vi "Main.vi"(7 "sweep rate, /min":dbl=0.2, 8 "sweep to:":dbl=4.0, 9 "sweep":T8(radio)=enum."2636a_smub") -> ()   [LabVIEW 2021] (continued)
                n1738 = property on="MFLI1_d3" class="Bool (strict)"() -> ("Value"=w2268:bool)  [unwired: 2 in, 2 out]
                n1739 = property on="data_caption" class="Str"() -> ("Value"=w2272:string)  [unwired: 2 in, 2 out]
                n1740 = property on="Figure_axis" class="Arr (strict)"() -> ("Value"=w2270:string[])  [unwired: 2 in, 2 out]
                n1741 = case shown="True" w2268 {
                  tunnel: w2272 -> [w2274 w2282]
                  tunnel: [w2274 w2281] -> w2271
                  tunnel: w2270 -> [w2273 w2280]
                  tunnel: [w2273 w2279] -> w2269
                  frame False {
                    # "not measure 2461 voltage (2461_meas_v)"
                  }
                  frame True {
                    w2277 = "MFLI1_d3_y"
                    w2278 = "MFLI1_d3_x"
                    w2276 = "\t"
                    w2275 = "MFLI1_d3_freq"
                    n1742 = Build Array (concatenate)(w2280, w2278, w2277, w2275) -> (w2279:string[])
                    n1743 = Concatenate Strings(w2282, w2278, w2276, w2277, w2276, w2275, w2276) -> (w2281:string)
                  }
                }
                n1744 = property on="Figure_axis" class="Arr (strict)"("Value"=w2269) -> ()  [unwired: 2 in, 2 out]
                n1745 = property on="data_caption" class="Str"("Value"=w2271) -> ()  [unwired: 2 in, 2 out]
              }
              frame #55 {
                # "MFLI_V"
                n1746 = property on="MFLI2_d3" class="Bool (strict)"() -> ("Value"=w2283:bool)  [unwired: 2 in, 2 out]
                n1747 = property on="data_caption" class="Str"() -> ("Value"=w2287:string)  [unwired: 2 in, 2 out]
                n1748 = property on="Figure_axis" class="Arr (strict)"() -> ("Value"=w2285:string[])  [unwired: 2 in, 2 out]
                n1749 = case shown="True" w2283 {
                  tunnel: w2287 -> [w2289 w2297]
                  tunnel: [w2289 w2296] -> w2286
                  tunnel: w2285 -> [w2288 w2295]
                  tunnel: [w2288 w2294] -> w2284
                  frame False {
                    # "not measure 2461 voltage (2461_meas_v)"
                  }
                  frame True {
                    w2292 = "MFLI2_d3_y"
                    w2293 = "MFLI2_d3_x"
                    w2291 = "\t"
                    w2290 = "MFLI2_d3_freq"
                    n1750 = Build Array (concatenate)(w2295, w2293, w2292, w2290) -> (w2294:string[])
                    n1751 = Concatenate Strings(w2297, w2293, w2291, w2292, w2291, w2290, w2291) -> (w2296:string)
                  }
                }
                n1752 = property on="Figure_axis" class="Arr (strict)"("Value"=w2284) -> ()  [unwired: 2 in, 2 out]
                n1753 = property on="data_caption" class="Str"("Value"=w2286) -> ()  [unwired: 2 in, 2 out]
              }
              frame #56 {
                # "MFLI_V"
                n1754 = property on="MFLI3_d3" class="Bool (strict)"() -> ("Value"=w2298:bool)  [unwired: 2 in, 2 out]
                n1755 = property on="data_caption" class="Str"() -> ("Value"=w2302:string)  [unwired: 2 in, 2 out]
                n1756 = property on="Figure_axis" class="Arr (strict)"() -> ("Value"=w2300:string[])  [unwired: 2 in, 2 out]
                n1757 = case shown="True" w2298 {
                  tunnel: w2302 -> [w2304 w2312]
                  tunnel: [w2304 w2311] -> w2301
                  tunnel: w2300 -> [w2303 w2310]
                  tunnel: [w2303 w2309] -> w2299
                  frame False {
                    # "not measure 2461 voltage (2461_meas_v)"
                  }
                  frame True {
                    w2307 = "MFLI3_d3_y"
                    w2308 = "MFLI3_d3_x"
                    w2306 = "\t"
                    w2305 = "MFLI3_d3_freq"
                    n1758 = Build Array (concatenate)(w2310, w2308, w2307, w2305) -> (w2309:string[])
                    n1759 = Concatenate Strings(w2312, w2308, w2306, w2307, w2306, w2305, w2306) -> (w2311:string)
                  }
                }
                n1760 = property on="Figure_axis" class="Arr (strict)"("Value"=w2299) -> ()  [unwired: 2 in, 2 out]
                n1761 = property on="data_caption" class="Str"("Value"=w2301) -> ()  [unwired: 2 in, 2 out]
              }
              frame #57 {
                # "MFLI_V"
                n1762 = property on="MFLI4_d3" class="Bool (strict)"() -> ("Value"=w2313:bool)  [unwired: 2 in, 2 out]
                n1763 = property on="data_caption" class="Str"() -> ("Value"=w2317:string)  [unwired: 2 in, 2 out]
                n1764 = property on="Figure_axis" class="Arr (strict)"() -> ("Value"=w2315:string[])  [unwired: 2 in, 2 out]
                n1765 = case shown="True" w2313 {
                  tunnel: w2317 -> [w2319 w2327]
                  tunnel: [w2319 w2326] -> w2316
                  tunnel: w2315 -> [w2318 w2325]
                  tunnel: [w2318 w2324] -> w2314
                  frame False {
                    # "not measure 2461 voltage (2461_meas_v)"
                  }
                  frame True {
                    w2322 = "MFLI4_d3_y"
                    w2323 = "MFLI4_d3_x"
                    w2321 = "\t"
                    w2320 = "MFLI4_d3_freq"
                    n1766 = Build Array (concatenate)(w2325, w2323, w2322, w2320) -> (w2324:string[])
                    n1767 = Concatenate Strings(w2327, w2323, w2321, w2322, w2321, w2320, w2321) -> (w2326:string)
                  }
                }
                n1768 = property on="Figure_axis" class="Arr (strict)"("Value"=w2314) -> ()  [unwired: 2 in, 2 out]
                n1769 = property on="data_caption" class="Str"("Value"=w2316) -> ()  [unwired: 2 in, 2 out]
              }
              frame #58 {
                # "MFLI_V"
                n1770 = property on="MFLI1_AuxOut0" class="Bool (strict)"() -> ("Value"=w2328:bool)  [unwired: 2 in, 2 out]
                n1771 = property on="data_caption" class="Str"() -> ("Value"=w2332:string)  [unwired: 2 in, 2 out]
                n1772 = property on="Figure_axis" class="Arr (strict)"() -> ("Value"=w2330:string[])  [unwired: 2 in, 2 out]
                n1773 = case shown="True" w2328 {
                  tunnel: w2332 -> [w2334 w2336]
                  tunnel: [w2334 w2337] -> w2331
                  tunnel: w2330 -> [w2333 w2335]
                  tunnel: [w2333 w2338] -> w2329
                  frame False {
                    # "not measure 2461 voltage (2461_meas_v)"
                  }
                  frame True {
                    w2339 = "MF1_AuxOut0"
                    n1774 = Build Array (concatenate)(w2335, w2339) -> (w2338:string[])
                    n1775 = Concatenate Strings(w2336, w2339, "\t") -> (w2337:string)
                  }
                }
                n1776 = property on="Figure_axis" class="Arr (strict)"("Value"=w2329) -> ()  [unwired: 2 in, 2 out]
                n1777 = property on="data_caption" class="Str"("Value"=w2331) -> ()  [unwired: 2 in, 2 out]
              }
            }
          }
          frame #2 {
            # "1 = 2400 1\n2 = 2400 2\n3 = 2400 3\n4 = 2636a smua\n5 = 2636a smub\n6 = do not sweep, just time\n7 = Teslatron_iPS_Field\n8 = Teslatron_iTC_Sample T"
            n1778 = property on="sweep" class="RadioBtnsControl (strict)"() -> ("Value"=w2341:T8)  [unwired: 2 in, 2 out]
            n1779 = case "reads current value from instrument which will be sweeping" shown="\"AuxOut0\"" w2341 {
              tunnel: [w2343 w2353 w2362 w2371 w2375 0.0 ("Measuremet") w2381 w2402 w2404 w2406] -> w2342
              frame "2400_1", Default {
                # "reads the voltage on 2400 1"
                n1780 = local read "2400 1 addr"() -> (w2347:u8)
                n1781 = Number To Decimal String(number=w2347) -> (decimal integer string=w2348:string)  [unwired: 1 in]
                n1782 = GPIB Write(0:w2348, 1:":READ?") -> (6:w2344:errorcluster)  [unwired: 3 in, 1 out]
                n1783 = GPIB Read(0:w2348, 1:3200, 3:w2344) -> (5:w2350:string)  [unwired: 2 in, 2 out]
                n1784 = String Subset(string=w2350, length (rest)=13) -> (substring=w2351:string)  [unwired: 1 in]
                n1785 = Fract/Exp String To Number(string=w2351) -> (number=w2343:dbl)  [unwired: 3 in, 1 out]
              }
              frame "2400_2" {
                # "reads the current on 2400 2"
                n1786 = local read "2400 2 addr"() -> (w2357:u8)
                n1787 = Number To Decimal String(number=w2357) -> (decimal integer string=w2358:string)  [unwired: 1 in]
                n1788 = GPIB Write(0:w2358, 1:":READ?") -> (6:w2354:errorcluster)  [unwired: 3 in, 1 out]
                n1789 = GPIB Read(0:w2358, 1:3200, 3:w2354) -> (5:w2360:string)  [unwired: 2 in, 2 out]
                n1790 = String Subset(string=w2360, offset (0)=14, length (rest)=13) -> (substring=w2361:string)
                n1791 = Fract/Exp String To Number(string=w2361) -> (number=w2353:dbl)  [unwired: 3 in, 1 out]
              }
              frame "2400_3" {
                # "reads the voltage on 2400 3"
                n1792 = local read "2400 3 addr"() -> (w2366:u8)
                n1793 = Number To Decimal String(number=w2366) -> (decimal integer string=w2367:string)  [unwired: 1 in]
                n1794 = GPIB Write(0:w2367, 1:":READ?") -> (6:w2363:errorcluster)  [unwired: 3 in, 1 out]
                n1795 = GPIB Read(0:w2367, 1:3200, 3:w2363) -> (5:w2369:string)  [unwired: 2 in, 2 out]
                n1796 = String Subset(string=w2369, length (rest)=13) -> (substring=w2370:string)  [unwired: 1 in]
                n1797 = Fract/Exp String To Number(string=w2370) -> (number=w2362:dbl)  [unwired: 3 in, 1 out]
              }
              frame "2636a_smua" {
                # "reads the voltage on 2636a smua"
                n1798 = local read "2614A addr"() -> (w2374:refnum<visa-resource-name>)
                n1799 = call "SinglePointMeasurement.vi"("Measure"=Measure."Voltage", "Channel"=Channel."a", "VISA resource name 2"=w2374) -> ("Measuremet"=w2371:dbl)  [unwired: 3 in, 4 out]
              }
              frame "2636a_smub" {
                # "reads the voltage on 2636a smub"
                n1800 = local read "2614A addr"() -> (w2378:refnum<visa-resource-name>)
                n1801 = call "SinglePointMeasurement.vi"("Measure"=Measure."Voltage", "Channel"=Channel."b", "VISA resource name 2"=w2378) -> ("Measuremet"=w2375:dbl)  [unwired: 3 in, 4 out]
              }
              frame "time_sweep" {
              }
              frame "iPS" {
                n1802 = property on="Sweep B" class="Bool (strict)"() -> ("Value"=w2380:bool)  [unwired: 2 in, 2 out]
                n1803 = case shown="False" w2380 {
                  tunnel: [w2382 w2400] -> w2381
                  frame False {
                    n1804 = stacked-sequence {
                      tunnel: [_ _ w2389 _] -> w2382
                      frame #0 {
                        n1805 = local read "iPS_addr_sweep"() -> (w2385:refnum<visa-resource-name>)
                        n1806 = property on="sweep to:" class="DigNum (strict)"() -> ("Value"=w2383:dbl)  [unwired: 2 in, 2 out]
                        n1807 = call "iPSset.vi"("Target Field, T"=w2383, "iPSSetCtrl"=iPSsetCtrl."Set Target Field", "VISA resource name"=w2385) -> ()  [unwired: 5 in, 4 out]
                      }
                      frame #1 {
                        n1808 = local read "iPS_addr_sweep"() -> (w2388:refnum<visa-resource-name>)
                        n1809 = property on="sweep rate, /min" class="DigNum (strict)"() -> ("Value"=w2386:dbl)  [unwired: 2 in, 2 out]
                        n1810 = call "iPSset.vi"("Field Rate, T/min"=w2386, "iPSSetCtrl"=iPSsetCtrl."Set Target Field Rate", "VISA resource name"=w2388) -> ()  [unwired: 5 in, 4 out]
                      }
                      frame #2 {
                        n1811 = property on="iPS_addr_sweep" class="VISAName"() -> ("Value"=w2391:refnum<visa-resource-name>)  [unwired: 2 in, 2 out]
                        n1812 = call "iPSread.vi"("iPSreadCtrl"=iPSreadCtrl."OutputField", "VISA resource name"=w2391) -> ("number"=w2389:dbl)  [unwired: 6 in, 3 out]
                      }
                      frame #3 {
                        n1813 = property on="sweep to:" class="DigNum (strict)"() -> ("Value"=w2392:dbl)  [unwired: 2 in, 2 out]
                        n1814 = Not Equal To 0?(x=w2392) -> (x != 0?=w2395:bool)
                        n1815 = local read "iPS_addr_sweep"() -> (w2397:refnum<visa-resource-name>)
                        n1816 = Select(t=iPSsetCtrl."Go to Field" ("iPSSetCtrl"), s=w2395, f=iPSsetCtrl."Go to Field" ("iPSSetCtrl")) -> (s? t:f=w2393:T16)
                        n1817 = call "iPSset.vi"("iPSSetCtrl"=w2393, "VISA resource name"=w2397) -> ()  [unwired: 6 in, 4 out]
                      }
                    }
                  }
                  frame True {
                    # "Measure magnetic field on IPS120-0"
                    n1818 = property on="iPS_addr_sweep" class="VISAName"() -> ("Value"=w2399:refnum<visa-resource-name>)  [unwired: 2 in, 2 out]
                    n1819 = call "iPSread.vi"("iPSreadCtrl"=iPSreadCtrl."OutputField", "VISA resource name"=w2399) -> ("number"=w2400:dbl)  [unwired: 6 in, 3 out]
                  }
                }
              }
              frame "iTC" {
                n1820 = property on="iPS_addr_sweep" class="VISAName"() -> ("Value"=w2401:refnum<visa-resource-name>)  [unwired: 2 in, 2 out]
                n1821 = call "iTCread.vi"("VISA resource name"=w2401, "iTCreadCtrl"=iTCreadCtrl."Sample Temp") -> ("number"=w2402:dbl)  [unwired: 5 in, 3 out]
              }
              frame "2461" {
                n1822 = property on="2461_addr_sweep" class="VISAName"() -> ("Value"=w2405:refnum<visa-resource-name>)  [unwired: 2 in, 2 out]
                n1823 = call <instrlib>:"Get Source Level.vi"("VISA resource name"=w2405) -> ("Current Level Out"=w2404:dbl)  [unwired: 7 in, 3 out]
              }
              frame "AuxOut0" {
                n1824 = property on="HandleOut" class="Clust (strict)"() -> ("Value"=w2408:T1)  [unwired: 2 in, 2 out]
                n1825 = call "MFLIcontrol.vi"("MFLI function"=MFLIcommand."Get AuxOut0", "handle in"=w2408) -> ("AuxOut0_Ampl"=w2406:dbl)  [unwired: 5 in, 4 out]
              }
            }
          }
          frame #3 {
            n1826 = property on="Linetrace or Mapping?" class="Bool (strict)"() -> ("Value"=w2409:bool)  [unwired: 2 in, 2 out]
            n1827 = case shown="True" w2409 {
              frame False {
                # "Reserve a name for new linetrace data file:"
                n1828 = property on="Data Folder" class="Path"() -> ("Value"=w2417:path)  [unwired: 2 in, 2 out]
                n1829 = call "AutoNamerDatExtraArtem.vi"("SweepType"="linetraces", "Custom User Path"=w2417) -> ("String"=w2415:string, "Path"=w2416:path)  [unwired: 2 in]
                n1830 = Path To String(path=w2416) -> (string=w2414:string)
                n1831 = Concatenate Strings(w2414, "\\", w2415) -> (w2413:string)
                n1832 = String To Path(string=w2413) -> (path=w2412:path)
                n1833 = local write "Data file:"(w2412) -> ()
              }
              frame True {
                n1834 = property on="Sweep Direction" class="Str"() -> ("Value"=w2418:string)  [unwired: 2 in, 2 out]
                n1835 = case shown="\"Sweep Down\"" w2418 {
                  frame "Sweep Up" {
                    n1836 = property on="UpNameString" class="Str"() -> ("Value"=w2420:string)  [unwired: 2 in, 2 out]
                    n1837 = String To Path(string=w2420) -> (path=w2419:path)
                    n1838 = local write "Data file:"(w2419) -> ()
                  }
                  frame "Sweep Down" {
                    n1839 = property on="DownNameString" class="Str"() -> ("Value"=w2421:string)  [unwired: 2 in, 2 out]
                    n1840 = String To Path(string=w2421) -> (path=w2422:path)
                    n1841 = local write "Data file:"(w2422) -> ()
                  }
                  frame "Ramp Down", Default {
                  }
                }
              }
            }
          }
          frame #4 {
            # "add \"formula\" string to the axis rings"
            n1842 = property on="Figure_axis" class="Arr (strict)"() -> ("Value"=w2425:string[])  [unwired: 2 in, 2 out]
            n1843 = Build Array (concatenate)(w2425, "formula") -> (w2423:string[])
            n1844 = property on="Figure_axis" class="Arr (strict)"("Value"=w2423) -> ()  [unwired: 2 in, 2 out]
          }
          frame #5 {
            # "passes array to ring"
            n1845 = property on="SuperHyper" class="Bool (strict)"() -> ("Value"=w2426:bool)  [unwired: 2 in, 2 out]
            n1846 = case shown="True" w2426 {
              frame True {
                # "records the fist line into the both upa nd down data file\nwhen table index=0"
                n1847 = property on="Table Index" class="DigNum (strict)"() -> ("Value"=w2435:dbl)  [unwired: 2 in, 2 out]
                n1848 = property on="HyperLoop Index" class="DigNum (strict)"() -> ("Value"=w2436:dbl)  [unwired: 2 in, 2 out]
                n1849 = property on="SuperHyper_Index" class="DigNum (strict)"() -> ("Value"=w2430:dbl)  [unwired: 2 in, 2 out]
                n1850 = Equal To 0?(x=w2435) -> (x = 0?=w2433:bool)
                n1851 = Equal To 0?(x=w2436) -> (x = 0?=w2434:bool)
                n1852 = Equal To 0?(x=w2430) -> (x = 0?=w2429:bool)
                n1853 = And(x=w2434, y=w2433) -> (x .and. y?=w2432:bool)
                n1854 = And(x=w2432, y=w2429) -> (x .and. y?=w2431:bool)
                n1855 = case shown="True" w2431 {
                  frame False {
                  }
                  frame True {
                    n1856 = property on="data_caption" class="Str"() -> ("Value"=w2440:string)  [unwired: 2 in, 2 out]
                    n1857 = local read "Data file:"() -> (w2437:path)
                    n1858 = Concatenate Strings(w2440, "\r") -> (w2439:string)
                    n1859 = Write to Text File(file (use dialog)=w2437, text=w2439) -> ()  [unwired: 2 in, 3 out]
                  }
                }
              }
              frame False {
                n1860 = property on="HyperLoop" class="Bool (strict)"() -> ("Value"=w2441:bool)  [unwired: 2 in, 2 out]
                n1861 = case shown="True" w2441 {
                  frame False {
                    n1862 = property on="Linetrace or Mapping?" class="Bool (strict)"() -> ("Value"=w2442:bool)  [unwired: 2 in, 2 out]
                    n1863 = case shown="True" w2442 {
                      frame False {
                        # "records the fist line into the data file"
                        n1864 = property on="data_caption" class="Str"() -> ("Value"=w2444:string)  [unwired: 2 in, 2 out]
                        n1865 = local read "Data file:"() -> (w2445:path)
                        n1866 = Concatenate Strings(w2444, "\r") -> (w2446:string)
                        n1867 = Write to Text File(file (use dialog)=w2445, text=w2446) -> ()  [unwired: 2 in, 3 out]
                      }
                      frame True {
                        # "records the fist line into the both upa nd down data file\nwhen table index=0"
                        n1868 = property on="Table Index" class="DigNum (strict)"() -> ("Value"=w2448:dbl)  [unwired: 2 in, 2 out]
                        n1869 = Equal To 0?(x=w2448) -> (x = 0?=w2447:bool)
                        n1870 = case shown="True" w2447 {
                          frame False {
                          }
                          frame True {
                            n1871 = property on="data_caption" class="Str"() -> ("Value"=w2452:string)  [unwired: 2 in, 2 out]
                            n1872 = local read "Data file:"() -> (w2449:path)
                            n1873 = Concatenate Strings(w2452, "\r") -> (w2451:string)
                            n1874 = Write to Text File(file (use dialog)=w2449, text=w2451) -> ()  [unwired: 2 in, 3 out]
                          }
                        }
                      }
                    }
                  }
                  frame True {
                    # "records the fist line into the both upa nd down data file\nwhen table index=0"
                    n1875 = property on="Table Index" class="DigNum (strict)"() -> ("Value"=w2456:dbl)  [unwired: 2 in, 2 out]
                    n1876 = property on="HyperLoop Index" class="DigNum (strict)"() -> ("Value"=w2457:dbl)  [unwired: 2 in, 2 out]
                    n1877 = Equal To 0?(x=w2456) -> (x = 0?=w2454:bool)
                    n1878 = Equal To 0?(x=w2457) -> (x = 0?=w2455:bool)
                    n1879 = And(x=w2455, y=w2454) -> (x .and. y?=w2453:bool)
                    n1880 = case shown="True" w2453 {
                      frame False {
                      }
                      frame True {
                        n1881 = property on="data_caption" class="Str"() -> ("Value"=w2461:string)  [unwired: 2 in, 2 out]
                        n1882 = local read "Data file:"() -> (w2458:path)
                        n1883 = Concatenate Strings(w2461, "\r") -> (w2460:string)
                        n1884 = Write to Text File(file (use dialog)=w2458, text=w2460) -> ()  [unwired: 2 in, 3 out]
                      }
                    }
                  }
                }
              }
            }
            n1885 = property on="Figure_axis" class="Arr (strict)"() -> ("Value"=w2428:string[])  [unwired: 2 in, 2 out]
            n1886 = property on="Xaxis" class="Ring (strict)"("Strings []"=w2428) -> ()  [unwired: 2 in, 2 out]
            n1887 = property on="Stop Sweep" class="Bool"("DisabledEnum"=T10."Enabled" ("Disabled")) -> ()  [unwired: 2 in, 2 out]
            n1888 = property on="Yright" class="Ring (strict)"("Strings []"=w2428) -> ()  [unwired: 2 in, 2 out]
            n1889 = property on="Yaxis" class="Ring (strict)"("Strings []"=w2428) -> ()  [unwired: 2 in, 2 out]
          }
        }
        n1890 = call "timeInSeconds.vi"() -> ("Numeric"=w1363:dbl)  [unwired: 2 in, 1 out]
        n1891 = while {
          shift-right: [w2537] -> _
          shift-left: w1362 -> [w2538]
          shift-right: [w2535] -> w1361
          shift-left: w1359 -> [w2534]
          tunnel: w1363 -> [w2532]
          stop <- w2525 stop-if-true
          # "initial value"
          # "Measure the selected channels"
          # "data array"
          # "this loop stops when target value is reached"
          # "error cluster to determine data flow"
          n1892 = stacked-sequence {
            tunnel: [_ _ w2559 _ _ _] -> w2526
            tunnel: [_ _ w2558 _ _ _] -> w2536
            tunnel: w2534 -> [_ _ w2552 _ _ _]
            tunnel: [w2544 _ _ _ _ _] -> w2533
            tunnel: w2532 -> [_ _ _ w2582 _ _]
            tunnel: [_ _ w2552 _ _ _] -> w2528
            tunnel: [_ _ _ _ _ w3348] -> w2524
            frame #0 {
              # "time is measured at the beginning\nand at the end of the cycle to\ncalculate delay time required to\nkeep set sweep rate"
              n1893 = flat-sequence {
                tunnel: [w2546] -> w2544
                frame #0 {
                  n1894 = property on="time delay, ms" class="DigNum (strict)"() -> ("Value"=w2545:dbl)  [unwired: 2 in, 2 out]
                  n1895 = Wait (ms)(milliseconds to wait=w2545) -> ()  [unwired: 1 out]
                }
                frame #1 {
                  n1896 = Tick Count (ms)() -> (millisecond timer value=w2546:u32)
                }
              }
            }
            frame #1 {
              w2547 = dbl[] []  # Empty array for data
              # "clear data array before each measurement cycle"
              n1897 = property on="data" class="Arr (strict)"("Value"=w2547) -> ()  [unwired: 2 in, 2 out]
            }
            frame #2 {
              # "add next sweep value to the data array"
              n1898 = property on="data" class="Arr (strict)"() -> ("Value"=w2557:dbl[])  [unwired: 2 in, 2 out]
              n1899 = property on="Sweep B" class="Bool (strict)"() -> ("Value"=w2549:bool)  [unwired: 2 in, 2 out]
              n1900 = local read "sweep"() -> (w2555:T8)
              n1901 = Not(x=w2549) -> (.not. x?=w2548:bool)
              n1902 = Equal?(x=w2555, y=T17."Radio Selection 7" ("sweep")) -> (x = y?=w2551:bool)
              n1903 = And(x=w2551, y=w2548) -> (x .and. y?=w2550:bool)
              n1904 = case shown="False" w2550 {
                tunnel: [w2566 w2578] -> w2559
                tunnel: [w2560 w2577] -> w2558
                tunnel: w2552 -> [_ w2575]
                tunnel: [w2560 w2575] -> w2553
                frame True {
                  n1905 = disable-structure shown="Disabled" {
                    disable-tunnel: [w2569 _] -> _
                    disable-tunnel: [w2568 _] -> _
                    frame Disabled {
                      n1906 = stacked-sequence {
                        tunnel: [_ w2571 _] -> w2569
                        tunnel: [_ _ w2573] -> w2568
                        frame #0 {
                          n1907 = local read "Hulk_SMS_addr"() -> (w2570:refnum<visa-resource-name>)
                          n1908 = VISA Clear(VISA resource name=w2570) -> ()  [unwired: 1 in, 2 out]
                        }
                        frame #1 {
                          # "acquires current output value"
                          n1909 = local read "Hulk_SMS_addr"() -> (w2572:refnum<visa-resource-name>)
                          n1910 = call "SMS_GET_OUTPUT.vi"("Hulk_SMS_addr"=w2572) -> ("Numeric"=w2571:dbl)  [unwired: 1 in, 2 out]
                        }
                        frame #2 {
                          # "checks, wheter ramp was finished"
                          n1911 = local read "Hulk_SMS_addr"() -> (w2574:refnum<visa-resource-name>)
                          n1912 = call "SMS_RAMP_STATUS.vi"("Hulk_SMS_addr"=w2574) -> ("selection"=w2573:bool)  [unwired: 1 in, 2 out]
                        }
                      }
                    }
                    frame Enabled {
                    }
                  }
                  n1913 = property on="iPS_addr_sweep" class="VISAName"() -> ("Value"=w2562:refnum<visa-resource-name>)  [unwired: 2 in, 2 out]
                  n1914 = property on="sweep to:" class="DigNum (strict)"() -> ("Value"=w2567:dbl)  [unwired: 2 in, 2 out]
                  n1915 = call "iPSread.vi"("iPSreadCtrl"=iPSreadCtrl."MagnetField", "VISA resource name"=w2562) -> ("number"=w2560:dbl)  [unwired: 6 in, 3 out]
                  n1916 = property on="Tolerance_Sweep" class="DigNum (strict)"() -> ("Value"=w2563:dbl)  [unwired: 2 in, 2 out]
                  n1917 = Subtract(x=w2560, y=w2567) -> (x-y=w2565:dbl)
                  n1918 = Absolute Value(x=w2565) -> (abs(x)=w2564:dbl)
                  n1919 = Less Or Equal?(x=w2564, y=w2563) -> (x <= y?=w2566:bool)
                }
                frame False {
                  # "calculate next value"
                  n1920 = call "CalculateNextValue.vi"("Target a 2"="sweep to:", "Channel a source value"=w2575, "Ch a sweep rate units/min"="sweep rate, /min", "time between points, sec"="time/point, sec", "Source a"=Source."Voltage") -> ("Target a"=w2577:dbl, "Boolean"=w2578:bool)
                }
              }
              n1921 = Build Array (concatenate)(w2557, w2553) -> (w2556:dbl[])
              n1922 = property on="data" class="Arr (strict)"("Value"=w2556) -> ()  [unwired: 2 in, 2 out]
            }
            frame #3 {
              n1923 = stacked-sequence "measurement sequence" {
                tunnel: w2582 -> [_ _ _ _ _ _ _ _ _ _ _ _ _ _ _ _ _ _ _ _ _ _ _ _ _ _ _ _ w2982 _ _ _ _ _ _ _ _ _ _ _ _ _ _ _ _ _ _ _ _ _ _ _ _ _ _ _ _ _ _]
                frame #0 {
                  # "check if in-phase\nsignal on lock-in 1 \nis to be measured"
                  n1924 = property on="data" class="Arr (strict)"() -> ("Value"=w2584:dbl[])  [unwired: 2 in, 2 out]
                  n1925 = local read "SR830 1 ip"() -> (w2583:bool)
                  n1926 = case shown="True" w2583 {
                    tunnel: w2584 -> [w2586 w2595]
                    tunnel: [w2586 w2594] -> w2585
                    frame False {
                      # "we are not measuring in phase signal on lock-in 1 (SR830_1_ip)"
                    }
                    frame True {
                      # "we are  measuring lock-in 1, in phase (SR830_1_ip)"
                      n1927 = local read "SR830 1 addr"() -> (w2588:u8)
                      n1928 = Number To Decimal String(number=w2588) -> (decimal integer string=w2587:string)  [unwired: 1 in]
                      n1929 = GPIB Write(0:w2587, 1:"OUTR?1") -> (6:w2593:errorcluster)  [unwired: 3 in, 1 out]
                      n1930 = GPIB Read(0:w2587, 1:3200, 3:w2593) -> (5:w2591:string)  [unwired: 2 in, 2 out]
                      n1931 = Fract/Exp String To Number(string=w2591) -> (number=w2590:dbl)  [unwired: 3 in, 1 out]
                      n1932 = Build Array (concatenate)(w2595, w2590) -> (w2594:dbl[])
                    }
                  }
                  n1933 = property on="data" class="Arr (strict)"("Value"=w2585) -> ()  [unwired: 2 in, 2 out]
                }
                frame #1 {
                  # "check if out-of-phase\nsignal on lock-in 1 \nis to be measured"
                  n1934 = property on="data" class="Arr (strict)"() -> ("Value"=w2597:dbl[])  [unwired: 2 in, 2 out]
                  n1935 = local read "SR830 1 oop"() -> (w2596:bool)
                  n1936 = case shown="True" w2596 {
                    tunnel: w2597 -> [w2599 w2608]
                    tunnel: [w2599 w2607] -> w2598
                    frame False {
                      # "we are not measuring out of phase signal on lock-in 1 (SR830_1_oop)"
                    }
                    frame True {
                      # "we are  measuring lock-in 1, out of phase (SR830_1_oop)"
                      n1937 = local read "SR830 1 addr"() -> (w2601:u8)
                      n1938 = Number To Decimal String(number=w2601) -> (decimal integer string=w2600:string)  [unwired: 1 in]
                      n1939 = GPIB Write(0:w2600, 1:"OUTR?2") -> (6:w2606:errorcluster)  [unwired: 3 in, 1 out]
                      n1940 = GPIB Read(0:w2600, 1:3200, 3:w2606) -> (5:w2604:string)  [unwired: 2 in, 2 out]
                      n1941 = Fract/Exp String To Number(string=w2604) -> (number=w2603:dbl)  [unwired: 3 in, 1 out]
                      n1942 = Build Array (concatenate)(w2608, w2603) -> (w2607:dbl[])
                    }
                  }
                  n1943 = property on="data" class="Arr (strict)"("Value"=w2598) -> ()  [unwired: 2 in, 2 out]
                }
                frame #2 {
                  # "check if in-phase\nsignal on lock-in 2 \nis to be measured"
                  n1944 = property on="data" class="Arr (strict)"() -> ("Value"=w2610:dbl[])  [unwired: 2 in, 2 out]
                  n1945 = local read "SR830 2 ip"() -> (w2609:bool)
                  n1946 = case shown="True" w2609 {
                    tunnel: w2610 -> [w2612 w2621]
                    tunnel: [w2612 w2620] -> w2611
                    frame False {
                      # "we are not measuring in phase signal on lock-in 2 (SR830_2_ip)"
                    }
                    frame True {
                      # "we are  measuring lock-in 2, in phase (SR830_2_ip)"
                      n1947 = local read "SR830 2 addr"() -> (w2614:u8)
                      n1948 = Number To Decimal String(number=w2614) -> (decimal integer string=w2613:string)  [unwired: 1 in]
                      n1949 = GPIB Write(0:w2613, 1:"OUTP?1") -> (6:w2619:errorcluster)  [unwired: 3 in, 1 out]
                      n1950 = GPIB Read(0:w2613, 1:3200, 3:w2619) -> (5:w2617:string)  [unwired: 2 in, 2 out]
                      n1951 = Fract/Exp String To Number(string=w2617) -> (number=w2616:dbl)  [unwired: 3 in, 1 out]
                      n1952 = Build Array (concatenate)(w2621, w2616) -> (w2620:dbl[])
                    }
                  }
                  n1953 = property on="data" class="Arr (strict)"("Value"=w2611) -> ()  [unwired: 2 in, 2 out]
                }
                frame #3 {
                  # "check if out-of-phase\nsignal on lock-in 2 \nis to be measured"
                  n1954 = property on="data" class="Arr (strict)"() -> ("Value"=w2623:dbl[])  [unwired: 2 in, 2 out]
                  n1955 = local read "SR830 2 oop"() -> (w2622:bool)
                  n1956 = case shown="True" w2622 {
                    tunnel: w2623 -> [w2625 w2634]
                    tunnel: [w2625 w2633] -> w2624
                    frame False {
                      # "we are not measuring out of phase signal on lock-in 2 (SR830_2_oop)"
                    }
                    frame True {
                      # "we are  measuring lock-in 2, out of phase (SR830_2_oop)"
                      n1957 = local read "SR830 2 addr"() -> (w2627:u8)
                      n1958 = Number To Decimal String(number=w2627) -> (decimal integer string=w2626:string)  [unwired: 1 in]
                      n1959 = GPIB Write(0:w2626, 1:"OUTP?2") -> (6:w2632:errorcluster)  [unwired: 3 in, 1 out]
                      n1960 = GPIB Read(0:w2626, 1:3200, 3:w2632) -> (5:w2630:string)  [unwired: 2 in, 2 out]
                      n1961 = Fract/Exp String To Number(string=w2630) -> (number=w2629:dbl)  [unwired: 3 in, 1 out]
                      n1962 = Build Array (concatenate)(w2634, w2629) -> (w2633:dbl[])
                    }
                  }
                  n1963 = property on="data" class="Arr (strict)"("Value"=w2624) -> ()  [unwired: 2 in, 2 out]
                }
                frame #4 {
                  # "check if in-phase\nsignal on lock-in 3 \nis to be measured"
                  n1964 = property on="data" class="Arr (strict)"() -> ("Value"=w2636:dbl[])  [unwired: 2 in, 2 out]
                  n1965 = local read "SR830 3 ip"() -> (w2635:bool)
                  n1966 = case shown="True" w2635 {
                    tunnel: w2636 -> [w2638 w2647]
                    tunnel: [w2638 w2646] -> w2637
                    frame False {
                      # "we are not measuring in phase signal on lock-in 3 (SR830_3_ip)"
                    }
                    frame True {
                      # "we are  measuring lock-in 3, in phase (SR830_3_ip)"
                      n1967 = local read "SR830 3 addr"() -> (w2640:u8)
                      n1968 = Number To Decimal String(number=w2640) -> (decimal integer string=w2639:string)  [unwired: 1 in]
                      n1969 = GPIB Write(0:w2639, 1:"OUTP?1") -> (6:w2645:errorcluster)  [unwired: 3 in, 1 out]
                      n1970 = GPIB Read(0:w2639, 1:3200, 3:w2645) -> (5:w2643:string)  [unwired: 2 in, 2 out]
                      n1971 = Fract/Exp String To Number(string=w2643) -> (number=w2642:dbl)  [unwired: 3 in, 1 out]
                      n1972 = Build Array (concatenate)(w2647, w2642) -> (w2646:dbl[])
                    }
                  }
                  n1973 = property on="data" class="Arr (strict)"("Value"=w2637) -> ()  [unwired: 2 in, 2 out]
                }
                frame #5 {
                  # "check if out-of-phase\nsignal on lock-in 3 \nis to be measured"
                  n1974 = property on="data" class="Arr (strict)"() -> ("Value"=w2649:dbl[])  [unwired: 2 in, 2 out]
                  n1975 = local read "SR830 3 oop"() -> (w2648:bool)
                  n1976 = case shown="True" w2648 {
                    tunnel: w2649 -> [w2651 w2660]
                    tunnel: [w2651 w2659] -> w2650
                    frame False {
                      # "we are not measuring out of phase signal on lock-in 3 (SR830_3_oop)"
                    }
                    frame True {
                      # "we are  measuring lock-in 3, out of phase (SR830_3_oop)"
                      n1977 = local read "SR830 3 addr"() -> (w2653:u8)
                      n1978 = Number To Decimal String(number=w2653) -> (decimal integer string=w2652:string)  [unwired: 1 in]
                      n1979 = GPIB Write(0:w2652, 1:"OUTP?2") -> (6:w2658:errorcluster)  [unwired: 3 in, 1 out]
                      n1980 = GPIB Read(0:w2652, 1:3200, 3:w2658) -> (5:w2656:string)  [unwired: 2 in, 2 out]
                      n1981 = Fract/Exp String To Number(string=w2656) -> (number=w2655:dbl)  [unwired: 3 in, 1 out]
                      n1982 = Build Array (concatenate)(w2660, w2655) -> (w2659:dbl[])
                    }
                  }
                  n1983 = property on="data" class="Arr (strict)"("Value"=w2650) -> ()  [unwired: 2 in, 2 out]
                }
                frame #6 {
                  # "check if in-phase\nsignal on lock-in 4 \nis to be measured"
                  n1984 = property on="data" class="Arr (strict)"() -> ("Value"=w2662:dbl[])  [unwired: 2 in, 2 out]
                  n1985 = local read "SR830 4 ip"() -> (w2661:bool)
                  n1986 = case shown="True" w2661 {
                    tunnel: w2662 -> [w2664 w2673]
                    tunnel: [w2664 w2672] -> w2663
                    frame False {
                      # "we are not measuring in phase signal on lock-in 4 (SR830_4_ip)"
                    }
                    frame True {
                      # "we are  measuring lock-in 4, in phase (SR830_4_ip)"
                      n1987 = local read "SR830 4 addr"() -> (w2666:u8)
                      n1988 = Number To Decimal String(number=w2666) -> (decimal integer string=w2665:string)  [unwired: 1 in]
                      n1989 = GPIB Write(0:w2665, 1:"OUTP?1") -> (6:w2671:errorcluster)  [unwired: 3 in, 1 out]
                      n1990 = GPIB Read(0:w2665, 1:3200, 3:w2671) -> (5:w2669:string)  [unwired: 2 in, 2 out]
                      n1991 = Fract/Exp String To Number(string=w2669) -> (number=w2668:dbl)  [unwired: 3 in, 1 out]
                      n1992 = Build Array (concatenate)(w2673, w2668) -> (w2672:dbl[])
                    }
                  }
                  n1993 = property on="data" class="Arr (strict)"("Value"=w2663) -> ()  [unwired: 2 in, 2 out]
                }
                frame #7 {
                  # "check if out-of-phase\nsignal on lock-in 4 \nis to be measured"
                  n1994 = property on="data" class="Arr (strict)"() -> ("Value"=w2675:dbl[])  [unwired: 2 in, 2 out]
                  n1995 = local read "SR830 4 oop"() -> (w2674:bool)
                  n1996 = case shown="True" w2674 {
                    tunnel: w2675 -> [w2677 w2686]
                    tunnel: [w2677 w2685] -> w2676
                    frame False {
                      # "we are not measuring out of phase signal on lock-in 4 (SR830_4_oop)"
                    }
                    frame True {
                      # "we are  measuring lock-in 4, out of phase (SR830_4_oop)"
                      n1997 = local read "SR830 4 addr"() -> (w2679:u8)
                      n1998 = Number To Decimal String(number=w2679) -> (decimal integer string=w2678:string)  [unwired: 1 in]
                      n1999 = GPIB Write(0:w2678, 1:"OUTP?2") -> (6:w2684:errorcluster)  [unwired: 3 in, 1 out]
                      n2000 = GPIB Read(0:w2678, 1:3200, 3:w2684) -> (5:w2682:string)  [unwired: 2 in, 2 out]
                      n2001 = Fract/Exp String To Number(string=w2682) -> (number=w2681:dbl)  [unwired: 3 in, 1 out]
                      n2002 = Build Array (concatenate)(w2686, w2681) -> (w2685:dbl[])
                    }
                  }
                  n2003 = property on="data" class="Arr (strict)"("Value"=w2676) -> ()  [unwired: 2 in, 2 out]
                }
                frame #8 {
                  # "check if in-phase\nsignal on lock-in 5 \nis to be measured"
                  n2004 = property on="data" class="Arr (strict)"() -> ("Value"=w2688:dbl[])  [unwired: 2 in, 2 out]
                  n2005 = local read "SR830 5 ip"() -> (w2687:bool)
                  n2006 = case shown="True" w2687 {
                    tunnel: w2688 -> [w2690 w2699]
                    tunnel: [w2690 w2698] -> w2689
                    frame False {
                      # "we are not measuring in phase signal on lock-in 5 (SR830_5_ip)"
                    }
                    frame True {
                      # "we are  measuring lock-in 5 in phase (SR830_5_ip)"
                      n2007 = local read "SR830 5 addr"() -> (w2692:u8)
                      n2008 = Number To Decimal String(number=w2692) -> (decimal integer string=w2691:string)  [unwired: 1 in]
                      n2009 = GPIB Write(0:w2691, 1:"OUTP?1") -> (6:w2697:errorcluster)  [unwired: 3 in, 1 out]
                      n2010 = GPIB Read(0:w2691, 1:3200, 3:w2697) -> (5:w2695:string)  [unwired: 2 in, 2 out]
                      n2011 = Fract/Exp String To Number(string=w2695) -> (number=w2694:dbl)  [unwired: 3 in, 1 out]
                      n2012 = Build Array (concatenate)(w2699, w2694) -> (w2698:dbl[])
                    }
                  }
                  n2013 = property on="data" class="Arr (strict)"("Value"=w2689) -> ()  [unwired: 2 in, 2 out]
                }
                frame #9 {
                  # "check if out-of-phase\nsignal on lock-in 5 \nis to be measured"
                  n2014 = property on="data" class="Arr (strict)"() -> ("Value"=w2701:dbl[])  [unwired: 2 in, 2 out]
                  n2015 = local read "SR830 5 oop"() -> (w2700:bool)
                  n2016 = case shown="True" w2700 {
                    tunnel: w2701 -> [w2703 w2712]
                    tunnel: [w2703 w2711] -> w2702
                    frame False {
                      # "we are not measuring out of phase signal on lock-in 5 (SR830_5_oop)"
                    }
                    frame True {
                      # "we are  measuring lock-in 5 out of phase (SR830_5_oop)"
                      n2017 = local read "SR830 5 addr"() -> (w2705:u8)
                      n2018 = Number To Decimal String(number=w2705) -> (decimal integer string=w2704:string)  [unwired: 1 in]
                      n2019 = GPIB Write(0:w2704, 1:"OUTP?2") -> (6:w2710:errorcluster)  [unwired: 3 in, 1 out]
                      n2020 = GPIB Read(0:w2704, 1:3200, 3:w2710) -> (5:w2708:string)  [unwired: 2 in, 2 out]
                      n2021 = Fract/Exp String To Number(string=w2708) -> (number=w2707:dbl)  [unwired: 3 in, 1 out]
                      n2022 = Build Array (concatenate)(w2712, w2707) -> (w2711:dbl[])
                    }
                  }
                  n2023 = property on="data" class="Arr (strict)"("Value"=w2702) -> ()  [unwired: 2 in, 2 out]
                }
                frame #10 {
                  # "check if voltage \non 2400 SouceMeter 1\nis to be measured"
                  n2024 = property on="data" class="Arr (strict)"() -> ("Value"=w2714:dbl[])  [unwired: 2 in, 2 out]
                  n2025 = local read "2400 1 meas v"() -> (w2713:bool)
                  n2026 = case shown="True" w2713 {
                    tunnel: w2714 -> [w2716 w2727]
                    tunnel: [w2716 w2726] -> w2715
                    frame False {
                      # "we are not measuring 2400 1, voltage (2400_1_v)"
                    }
                    frame True {
                      # "we are  measuring 2400 1, voltage (2400_1_v)"
                      n2027 = local read "2400 1 addr"() -> (w2721:u8)
                      n2028 = Number To Decimal String(number=w2721) -> (decimal integer string=w2720:string)  [unwired: 1 in]
                      n2029 = GPIB Write(0:w2720, 1:":READ?") -> (6:w2725:errorcluster)  [unwired: 3 in, 1 out]
                      n2030 = GPIB Read(0:w2720, 1:3200, 3:w2725) -> (5:w2718:string)  [unwired: 2 in, 2 out]
                      n2031 = String Subset(string=w2718, length (rest)=13) -> (substring=w2717:string)  [unwired: 1 in]
                      n2032 = Fract/Exp String To Number(string=w2717) -> (number=w2723:dbl)  [unwired: 3 in, 1 out]
                      n2033 = Build Array (concatenate)(w2727, w2723) -> (w2726:dbl[])
                    }
                  }
                  n2034 = property on="data" class="Arr (strict)"("Value"=w2715) -> ()  [unwired: 2 in, 2 out]
                }
                frame #11 {
                  # "check if current \non 2400 SouceMeter 1\nis to be measured"
                  n2035 = property on="data" class="Arr (strict)"() -> ("Value"=w2729:dbl[])  [unwired: 2 in, 2 out]
                  n2036 = local read "2400 1 meas i"() -> (w2728:bool)
                  n2037 = case shown="True" w2728 {
                    tunnel: w2729 -> [w2731 w2743]
                    tunnel: [w2731 w2742] -> w2730
                    frame False {
                      # "we are not measuring 2400 1, current (2400_1_i)"
                    }
                    frame True {
                      # "we are  measuring 2400 1, current (2400_1_i)"
                      n2038 = local read "2400 1 addr"() -> (w2737:u8)
                      n2039 = Number To Decimal String(number=w2737) -> (decimal integer string=w2736:string)  [unwired: 1 in]
                      n2040 = GPIB Write(0:w2736, 1:":READ?") -> (6:w2741:errorcluster)  [unwired: 3 in, 1 out]
                      n2041 = GPIB Read(0:w2736, 1:3200, 3:w2741) -> (5:w2734:string)  [unwired: 2 in, 2 out]
                      n2042 = String Subset(string=w2734, offset (0)=14, length (rest)=13) -> (substring=w2733:string)
                      n2043 = Fract/Exp String To Number(string=w2733) -> (number=w2739:dbl)  [unwired: 3 in, 1 out]
                      n2044 = Build Array (concatenate)(w2743, w2739) -> (w2742:dbl[])
                    }
                  }
                  n2045 = property on="data" class="Arr (strict)"("Value"=w2730) -> ()  [unwired: 2 in, 2 out]
                }
                frame #12 {
                  # "check if voltage \non 2400 SouceMeter 2\nis to be measured"
                  n2046 = property on="data" class="Arr (strict)"() -> ("Value"=w2745:dbl[])  [unwired: 2 in, 2 out]
                  n2047 = local read "2400 2 meas v"() -> (w2744:bool)
                  n2048 = case shown="True" w2744 {
                    tunnel: w2745 -> [w2747 w2758]
                    tunnel: [w2747 w2757] -> w2746
                    frame False {
                      # "we are not measuring 2400 2, voltage (2400_2_v)"
                    }
                    frame True {
                      # "we are  measuring 2400 2, voltage (2400_2_v)"
                      n2049 = local read "2400 2 addr"() -> (w2752:u8)
                      n2050 = Number To Decimal String(number=w2752) -> (decimal integer string=w2751:string)  [unwired: 1 in]
                      n2051 = GPIB Write(0:w2751, 1:":READ?") -> (6:w2756:errorcluster)  [unwired: 3 in, 1 out]
                      n2052 = GPIB Read(0:w2751, 1:3200, 3:w2756) -> (5:w2749:string)  [unwired: 2 in, 2 out]
                      n2053 = String Subset(string=w2749, length (rest)=13) -> (substring=w2748:string)  [unwired: 1 in]
                      n2054 = Fract/Exp String To Number(string=w2748) -> (number=w2754:dbl)  [unwired: 3 in, 1 out]
                      n2055 = Build Array (concatenate)(w2758, w2754) -> (w2757:dbl[])
                    }
                  }
                  n2056 = property on="data" class="Arr (strict)"("Value"=w2746) -> ()  [unwired: 2 in, 2 out]
                }
                frame #13 {
                  # "check if current \non 2400 SouceMeter 2\nis to be measured"
                  n2057 = property on="data" class="Arr (strict)"() -> ("Value"=w2760:dbl[])  [unwired: 2 in, 2 out]
                  n2058 = local read "2400 2 meas i"() -> (w2759:bool)
                  n2059 = case shown="True" w2759 {
                    tunnel: w2760 -> [w2762 w2774]
                    tunnel: [w2762 w2773] -> w2761
                    frame False {
                      # "we are not measuring 2400 2, current (2400_2_i)"
                    }
                    frame True {
                      # "we are  measuring 2400 2, current (2400_2_i)"
                      n2060 = local read "2400 2 addr"() -> (w2768:u8)
                      n2061 = Number To Decimal String(number=w2768) -> (decimal integer string=w2767:string)  [unwired: 1 in]
                      n2062 = GPIB Write(0:w2767, 1:":READ?") -> (6:w2772:errorcluster)  [unwired: 3 in, 1 out]
                      n2063 = GPIB Read(0:w2767, 1:3200, 3:w2772) -> (5:w2765:string)  [unwired: 2 in, 2 out]
                      n2064 = String Subset(string=w2765, offset (0)=14, length (rest)=13) -> (substring=w2764:string)
                      n2065 = Fract/Exp String To Number(string=w2764) -> (number=w2770:dbl)  [unwired: 3 in, 1 out]
                      n2066 = Build Array (concatenate)(w2774, w2770) -> (w2773:dbl[])
                    }
                  }
                  n2067 = property on="data" class="Arr (strict)"("Value"=w2761) -> ()  [unwired: 2 in, 2 out]
                }
                frame #14 {
                  # "check if voltage \non 2400 SouceMeter 3\nis to be measured"
                  n2068 = property on="data" class="Arr (strict)"() -> ("Value"=w2776:dbl[])  [unwired: 2 in, 2 out]
                  n2069 = local read "2400 3 meas v"() -> (w2775:bool)
                  n2070 = case shown="True" w2775 {
                    tunnel: w2776 -> [w2778 w2789]
                    tunnel: [w2778 w2788] -> w2777
                    frame False {
                      # "we are not measuring 2400 3, voltage (2400_3_v)"
                    }
                    frame True {
                      # "we are  measuring 2400 3, voltage (2400_3_v)"
                      n2071 = local read "2400 3 addr"() -> (w2783:u8)
                      n2072 = Number To Decimal String(number=w2783) -> (decimal integer string=w2782:string)  [unwired: 1 in]
                      n2073 = GPIB Write(0:w2782, 1:":READ?") -> (6:w2787:errorcluster)  [unwired: 3 in, 1 out]
                      n2074 = GPIB Read(0:w2782, 1:3200, 3:w2787) -> (5:w2780:string)  [unwired: 2 in, 2 out]
                      n2075 = String Subset(string=w2780, length (rest)=13) -> (substring=w2779:string)  [unwired: 1 in]
                      n2076 = Fract/Exp String To Number(string=w2779) -> (number=w2785:dbl)  [unwired: 3 in, 1 out]
                      n2077 = Build Array (concatenate)(w2789, w2785) -> (w2788:dbl[])
                    }
                  }
                  n2078 = property on="data" class="Arr (strict)"("Value"=w2777) -> ()  [unwired: 2 in, 2 out]
                }
                frame #15 {
                  # "check if current \non 2400 SouceMeter 3\nis to be measured"
                  n2079 = property on="data" class="Arr (strict)"() -> ("Value"=w2791:dbl[])  [unwired: 2 in, 2 out]
                  n2080 = local read "2400 3 meas i"() -> (w2790:bool)
                  n2081 = case shown="True" w2790 {
                    tunnel: w2791 -> [w2793 w2805]
                    tunnel: [w2793 w2804] -> w2792
                    frame False {
                      # "we are not measuring 2400 3, current (2400_3_i)"
                    }
                    frame True {
                      # "we are  measuring 2400 3, current (2400_3_i)"
                      n2082 = local read "2400 3 addr"() -> (w2799:u8)
                      n2083 = Number To Decimal String(number=w2799) -> (decimal integer string=w2798:string)  [unwired: 1 in]
                      n2084 = GPIB Write(0:w2798, 1:":READ?") -> (6:w2803:errorcluster)  [unwired: 3 in, 1 out]
                      n2085 = GPIB Read(0:w2798, 1:3200, 3:w2803) -> (5:w2796:string)  [unwired: 2 in, 2 out]
                      n2086 = String Subset(string=w2796, offset (0)=14, length (rest)=13) -> (substring=w2795:string)
                      n2087 = Fract/Exp String To Number(string=w2795) -> (number=w2801:dbl)  [unwired: 3 in, 1 out]
                      n2088 = Build Array (concatenate)(w2805, w2801) -> (w2804:dbl[])
                    }
                  }
                  n2089 = property on="data" class="Arr (strict)"("Value"=w2792) -> ()  [unwired: 2 in, 2 out]
                }
                frame #16 {
                  # "check if 1st channel \non Keithley 2182A 1\nis to be measured"
                  n2090 = property on="data" class="Arr (strict)"() -> ("Value"=w2807:dbl[])  [unwired: 2 in, 2 out]
                  n2091 = local read "2182A 1 ch1"() -> (w2806:bool)
                  n2092 = case shown="True" w2806 {
                    tunnel: w2807 -> [w2809 w2818]
                    tunnel: [w2809 w2817] -> w2808
                    frame False {
                      # "we are not measuring 2182A 1 channel 1 (2182A_1_ch1)"
                    }
                    frame True {
                      # "we are  measuring 2182A 1 channel 1 (2182A_1_ch1)"
                      n2093 = local read "2182A 1 addr"() -> (w2812:u8)
                      n2094 = Number To Decimal String(number=w2812) -> (decimal integer string=w2811:string)  [unwired: 1 in]
                      n2095 = GPIB Write(0:w2811, 1:":SENSe:DATA:FRES?") -> (6:w2816:errorcluster)  [unwired: 3 in, 1 out]
                      n2096 = GPIB Read(0:w2811, 1:200, 3:w2816) -> (5:w2810:string)  [unwired: 2 in, 2 out]
                      n2097 = Fract/Exp String To Number(string=w2810) -> (number=w2814:dbl)  [unwired: 3 in, 1 out]
                      n2098 = Build Array (concatenate)(w2818, w2814) -> (w2817:dbl[])
                    }
                  }
                  n2099 = property on="data" class="Arr (strict)"("Value"=w2808) -> ()  [unwired: 2 in, 2 out]
                }
                frame #17 {
                  # "check if 2nd channel \non Keithley 2182A 1\nis to be measured"
                  n2100 = property on="data" class="Arr (strict)"() -> ("Value"=w2820:dbl[])  [unwired: 2 in, 2 out]
                  n2101 = local read "2182A 1 ch2"() -> (w2819:bool)
                  n2102 = case shown="True" w2819 {
                    tunnel: w2820 -> [w2822 w2835]
                    tunnel: [w2822 w2834] -> w2821
                    frame False {
                      # "we are not measuring 2182A 1 channel 2 (2182A_1_ch2)"
                    }
                    frame True {
                      # "switching to channel 2 and then\nback to channel 1"
                      # "we are  measuring 2182A 1 channel 2 (2182A_1_ch2)"
                      n2103 = local read "2182A 1 addr"() -> (w2829:u8)
                      n2104 = Number To Decimal String(number=w2829) -> (decimal integer string=w2824:string)  [unwired: 1 in]
                      n2105 = GPIB Write(0:w2824, 1:":SENSe:CHAN 2") -> (6:w2826:errorcluster)  [unwired: 3 in, 1 out]
                      n2106 = GPIB Write(0:w2824, 1:":SENSe:DATA:FRES?", 3:w2826) -> (6:w2833:errorcluster)  [unwired: 2 in, 1 out]
                      n2107 = GPIB Read(0:w2824, 1:200, 3:w2833) -> (5:w2828:string, 7:w2825:errorcluster)  [unwired: 2 in, 1 out]
                      n2108 = GPIB Write(0:w2824, 1:":SENSe:CHAN 1", 3:w2825) -> ()  [unwired: 2 in, 2 out]
                      n2109 = Fract/Exp String To Number(string=w2828) -> (number=w2831:dbl)  [unwired: 3 in, 1 out]
                      n2110 = Build Array (concatenate)(w2835, w2831) -> (w2834:dbl[])
                    }
                  }
                  n2111 = property on="data" class="Arr (strict)"("Value"=w2821) -> ()  [unwired: 2 in, 2 out]
                }
                frame #18 {
                  # "check if 1st channel \non Keithley 2182A 2\nis to be measured"
                  n2112 = property on="data" class="Arr (strict)"() -> ("Value"=w2837:dbl[])  [unwired: 2 in, 2 out]
                  n2113 = local read "2182A 2 ch1"() -> (w2836:bool)
                  n2114 = case shown="True" w2836 {
                    tunnel: w2837 -> [w2839 w2848]
                    tunnel: [w2839 w2847] -> w2838
                    frame False {
                      # "we are not measuring 2182A 2 channel 1 (2182A_2_ch1)"
                    }
                    frame True {
                      # "we are  measuring 2182A 2 channel 1 (2182A_2_ch1)"
                      n2115 = local read "2182A 2 addr"() -> (w2842:u8)
                      n2116 = Number To Decimal String(number=w2842) -> (decimal integer string=w2841:string)  [unwired: 1 in]
                      n2117 = GPIB Write(0:w2841, 1:":SENSe:DATA:FRES?") -> (6:w2846:errorcluster)  [unwired: 3 in, 1 out]
                      n2118 = GPIB Read(0:w2841, 1:200, 3:w2846) -> (5:w2840:string)  [unwired: 2 in, 2 out]
                      n2119 = Fract/Exp String To Number(string=w2840) -> (number=w2844:dbl)  [unwired: 3 in, 1 out]
                      n2120 = Build Array (concatenate)(w2848, w2844) -> (w2847:dbl[])
                    }
                  }
                  n2121 = property on="data" class="Arr (strict)"("Value"=w2838) -> ()  [unwired: 2 in, 2 out]
                }
                frame #19 {
                  # "check if 2nd channel \non Keithley 2182A 2\nis to be measured"
                  n2122 = property on="data" class="Arr (strict)"() -> ("Value"=w2850:dbl[])  [unwired: 2 in, 2 out]
                  n2123 = local read "2182A 2 ch2"() -> (w2849:bool)
                  n2124 = case shown="True" w2849 {
                    tunnel: w2850 -> [w2852 w2865]
                    tunnel: [w2852 w2864] -> w2851
                    frame False {
                      # "we are not measuring 2182A 2 channel 2 (2182A_2_ch2)"
                    }
                    frame True {
                      # "switching to channel 2 and then\nback to channel 1"
                      # "we are  measuring 2182A 2 channel 2 (2182A_2_ch2)"
                      n2125 = local read "2182A 2 addr"() -> (w2859:u8)
                      n2126 = Number To Decimal String(number=w2859) -> (decimal integer string=w2854:string)  [unwired: 1 in]
                      n2127 = GPIB Write(0:w2854, 1:":SENSe:CHAN 2") -> (6:w2856:errorcluster)  [unwired: 3 in, 1 out]
                      n2128 = GPIB Write(0:w2854, 1:":SENSe:DATA:FRES?", 3:w2856) -> (6:w2863:errorcluster)  [unwired: 2 in, 1 out]
                      n2129 = GPIB Read(0:w2854, 1:200, 3:w2863) -> (5:w2858:string, 7:w2855:errorcluster)  [unwired: 2 in, 1 out]
                      n2130 = GPIB Write(0:w2854, 1:":SENSe:CHAN 1", 3:w2855) -> ()  [unwired: 2 in, 2 out]
                      n2131 = Fract/Exp String To Number(string=w2858) -> (number=w2861:dbl)  [unwired: 3 in, 1 out]
                      n2132 = Build Array (concatenate)(w2865, w2861) -> (w2864:dbl[])
                    }
                  }
                  n2133 = property on="data" class="Arr (strict)"("Value"=w2851) -> ()  [unwired: 2 in, 2 out]
                }
                frame #20 {
                  # "check if 1st channel \non Keithley 2182A 3\nis to be measured"
                  n2134 = property on="data" class="Arr (strict)"() -> ("Value"=w2867:dbl[])  [unwired: 2 in, 2 out]
                  n2135 = local read "2182A 3 ch1"() -> (w2866:bool)
                  n2136 = case shown="True" w2866 {
                    tunnel: w2867 -> [w2869 w2878]
                    tunnel: [w2869 w2877] -> w2868
                    frame False {
                      # "we are not measuring 2182A 3 channel 1 (2182A_3_ch1)"
                    }
                    frame True {
